vi "_tester2_.vi"() -> ()   [LabVIEW 2025]
uses:
  LabVIEWpcm.dll
panel:
  out "counrters":i32
  in  "Stop Button 2":bool
  out "sum":u8
  out "counter":i32
  out "Waveform Chart 4":u64(graph)
  out "Waveform Chart 3":dbl(graph)
  out "Waveform Chart 2":u64(graph)
  out "Waveform Chart":dbl(graph)
  out "l3miss":u64
  out "l3hit":dbl
  out "lv2miss":u64
  out "lv2hit":dbl
  out "init":i32
  out "return type":i32
  out "bytes":u64
  out "ipc":dbl
  # "MUST BE RUN AS ADMINISTRATOR!!!"
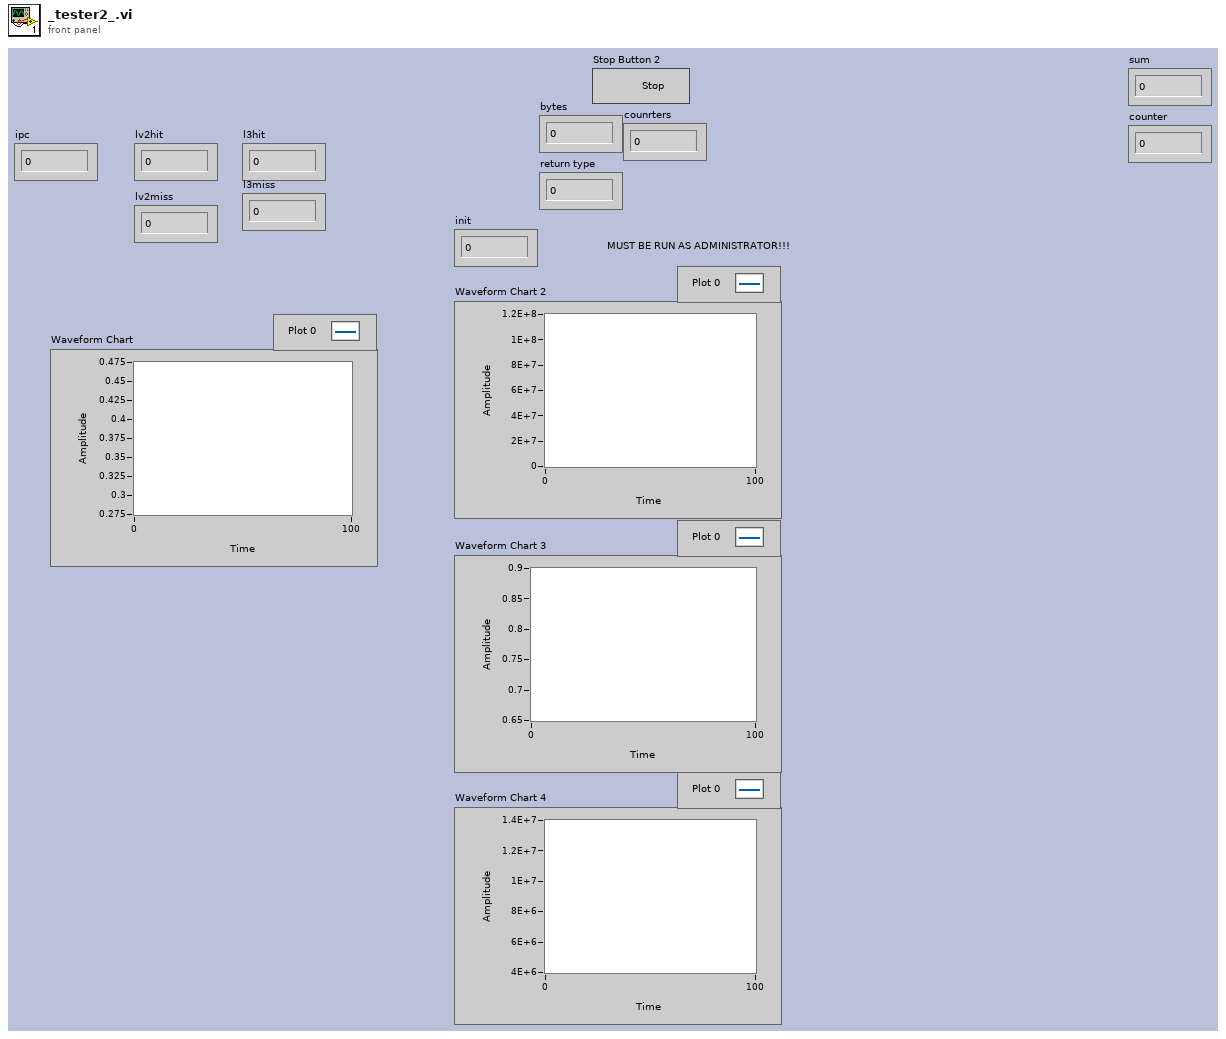
[diagram p1: front panel]
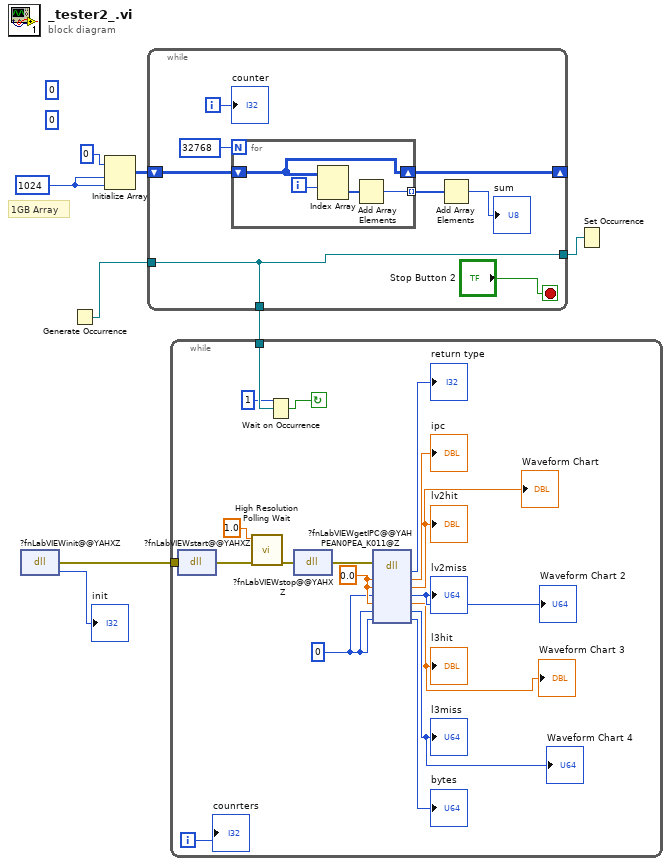
[diagram p0: block diagram]
diagram:
  (unwired) 0 ("Processor")
  (unwired) i64 0 ("Period")
  w5 = 1024 ("dimension size")
  # "1GB Array"
  n1 = dll-call lib="C:/Users/Andrey/Desktop/intel-pcm/build/x64/Release/LabVIEWpcm.dll" fn="?fnLabVIEWinit@@YAHXZ"() -> (error out=w8:errorcluster, "return type"=→"init":i32)  [unwired: 3 in, 1 out]
  n2 = Generate Occurrence() -> (w2:refnum<k4>)
  n3 = Initialize Array(u8 0, w5, w5) -> (w4:u8[][])
  n4 = while {
    shift-right: [w11] -> _
    shift-left: w4 -> [w14]
    tunnel: [w9] -> w3
    tunnel: w2 -> [w9]
    tunnel: [w9] -> w1
    i -> [w10]
    stop <- "Stop Button 2" stop-if-true
    n5 = for {
      N: 32768 ("dimension size") -> [_]
      tunnel: [w19] -> w13 mode=indexing
      shift-right: [w18] -> w11
      shift-left: w14 -> [w18]
      i -> [w17]
      n6 = Index Array(array=w18, index (row)=w17) -> (element=w20:u8[])  [unwired: 1 in]
      n7 = Add Array Elements(numeric array=w20) -> (sum=w19:u8)
    }
    n8 = Add Array Elements(numeric array=w13) -> (sum=→"sum":u8)
    "counter" <- w10
  }
  n9 = while {
    tunnel: w8 -> [w38]
    tunnel: w1 -> [w24]
    i -> [w21]
    stop <- w22 continue-if-true
    w29 = u64 0 ("bytes")
    w30 = 0.0 ("ipc")
    n10 = dll-call lib="C:/Users/Andrey/Desktop/intel-pcm/build/x64/Release/LabVIEWpcm.dll" fn="?fnLabVIEWstart@@YAHXZ"(error in=w38) -> (error out=w37:errorcluster)  [unwired: 3 in, 1 out]
    n11 = call <vilib>:"High Resolution Polling Wait.vi"("error in (no error)"=w37, "seconds to wait"=1.0) -> ("error out"=w36:errorcluster)  [unwired: 9 in]
    n12 = Wait on Occurrence(2:w24, 3:1 ("ms timeout (-1)")) -> (0:w22:bool)  [unwired: 1 in]
    n13 = dll-call lib="C:/Users/Andrey/Desktop/intel-pcm/build/x64/Release/LabVIEWpcm.dll" fn="?fnLabVIEWstop@@YAHXZ"(error in=w36) -> (error out=w35:errorcluster)  [unwired: 3 in, 1 out]
    n14 = dll-call lib="C:/Users/Andrey/Desktop/intel-pcm/build/x64/Release/LabVIEWpcm.dll" fn="?fnLabVIEWgetIPC@@YAHPEAN0PEA_K011@Z"(error in=w35, "ipc"=w30, "lv2hit"=w30, "lv2miss"=w29, "l3hit"=w30, "l3miss"=w29, "bytes"=w29) -> ("return type"=→"return type":i32, "ipc"=→"ipc":dbl, "lv2hit"=→"lv2hit" →"Waveform Chart":dbl, "lv2miss"=→"lv2miss" →"Waveform Chart 2":u64, "l3hit"=→"l3hit" →"Waveform Chart 3":dbl, "l3miss"=→"l3miss" →"Waveform Chart 4":u64, "bytes"=→"bytes":u64)  [unwired: 2 in, 2 out]
    "counrters" <- w21
  }
  n15 = Set Occurrence(w3) -> ()
